vi "Read Limits File_forTestStand use.vi"(11 "Limt_Filename":string="All_Test_Scripts") -> (3 "All_Limits":string[][](array[string])=[["TestName", "Key", "TestNumber", "Low Limit", "High Limit", "TestStand Test Name", "", "", ""], ["IVIOKGD", "Start", "1", "0", "3", "IVSU_LowPower_Initial", "", "", ""], ["", "End", "2", "50", "100", "IVSU_State0x00_Initial", "", "", ""], ["", "", "", "", "", "", "", "", "`"], ["Initial_States", "Start", "1", "50", "100", "IVSU_State0x0F_Initial", "", "", ""], ["", "End", "2", "50", "100", "IVSU_State0xF0_Initial", "", "", ""], ["", "", "", "", "", "", "", "", ""], ["Rfree_Initial", "Start", "1", "395k", "3M", "RF1", "", "", ""], ["", "", "2", "395k", "3M", "RF2", "", "", ""], ["", "", "3", "445k", "3M", "RF3", "", "", ""], ["", "End", "4", "445k", "3M", "RF4", "", "", ""], ["", "", "", "", "", "", "", "", ""], ["Ron_Initial", "Start", "1", "0.35", "2", "RF1", "", "", ""], ["", "", "2", "0.35", "2", "RF2", "", "", ""], ["", "", "3", "0.35", "2", "RF3", "", "", ""], ["", "End", "4", "0.35", "2", "RF4", "", "", ""], ["", "", "", "", "", "", "", "", ""], ["Ron_Conditioned", "Start", "1", "0.35", "1", "RF1", "", "", ""], ["", "", "2", "0.35", "1", "RF2", "", "", ""], ["", "", "3", "0.35", "1", "RF3", "", "", ""], ["", "End", "4", "0.35", "1", "RF4", "", "", ""], ["", "", "", "", "", "", "", "", ""], ["Butterfly", "Start", "55", "33", "39", "R_VPI", "", "", ""], ["", "End", "56", "30", "39", "R_VRL", "", "", ""], ["", "", "", "", "", "", "", "", ""], ["Rshunt", "Start", "1", "10", "20", "Rshunt_RF1", "", "", ""], ["", "", "2", "10", "20", "Rshunt_RF2", "", "", ""], ["", "", "3", "10", "20", "Rshunt_RF3", "", "", ""], ["", "End", "4", "10", "20", "Rshunt_RF4", "", "", ""], ["", "", "", "", "", "", "", "", ""], ["Guardian", "Start", "1", "1", "5", "GuardianPilot_On", "", "", ""], ["", "End", "2", "175k", "225k", "GuardianPilot_Off", "", "", ""], ["", "", "", "", "", "", "", "", ""], ["Final_States", "Start", "1", "50", "100", "IVSU_State0x0F_Final", "", "", ""], ["", "End", "2", "50", "100", "IVSU_State0xF0_Final", "", "", ""], ["", "", "", "", "", "", "", "", ""], ["Rfree_Final", "Start", "1", "395k", "445k", "RF1", "", "", ""], ["", "", "2", "395k", "445k", "RF2", "", "", ""], ["", "", "3", "445k", "495k", "RF3", "", "", ""], ["", "End", "4", "445k", "495k", "RF4", "", "", ""], ["", "", "", "", "", "", "", "", ""], ["", "", "", "", "", "", "", "", ""], ["Reverse_IVIOKGD", "Start", "1", "50", "100", "IVSU_State0x00_Final", "", "", ""], ["", "End", "2", "0", "3", "IVSU_LowPower_Final", "", "", ""]])   [LabVIEW 2013]
uses:
  <vilib>/Utility/file.llb/Read From Spreadsheet File (string).vi
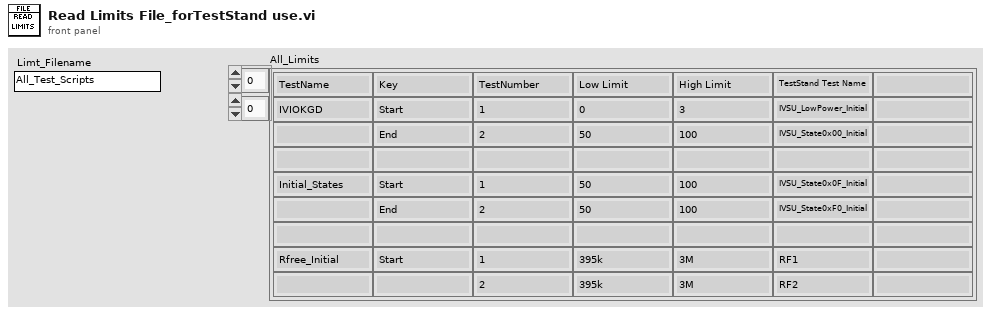
[diagram p1: front panel]
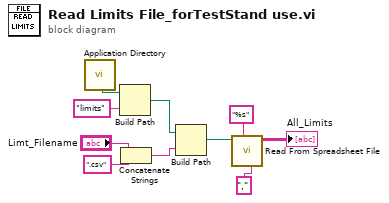
[diagram p0: block diagram]
diagram:
  n1 = call <vilib>:"Application Directory.vi"() -> ("Application Directory"=w4:path)
  n2 = Build Path(base path=w4, name or relative path="limits") -> (appended path=w2:path)
  n3 = Concatenate Strings("Limt_Filename", ".csv" ("string")) -> (w5:string)
  n4 = Build Path(base path=w2, name or relative path=w5) -> (appended path=w1:path)
  n5 = call-poly <vilib>:"Read From Spreadsheet File.vi"("delimiter (\\t)"="," ("delimiter (\\t)"), "format (%s)"="%s", "file path (dialog if empty)"=w1) -> ("all rows"=→"All_Limits":string[][])  [unwired: 4 in, 4 out]
